vi "Read Waveform.vi"(0 "CS++Scope":refnum<class "CS++Scope.lvclass">, 1 "channel name (\"CHANNEL1\")":string="CHANNEL1", 2 "maximum time (5000ms)":i32=5000, 3 "waveform size (0)":i32=1000 caption="waveform size (1000)", 5 "error in (no error)":errorcluster) -> (14 "CS++Scope out":refnum<class "CS++Scope.lvclass">, 15 "waveform array":dbl[unit][](array[numeric]) format="%.3f", 16 "actual points":i32, 17 "initial x":dbl[unit] caption="initial x (seconds)" format="%^.2e", 18 "x increment":dbl[unit] caption="x increment (seconds)" format="%^.2e", 19 "error out":errorcluster)   [LabVIEW 2016, in "CS++Scope.lvlib" / "CS++Scope.lvclass"]
doc: "This VI initiates an acquisition on all channels that you enable with the IviScope Configure Channel VI. If the channel you specify in the Channel Name parameter is not enabled for the acquisition, this VI returns the IVISCOPE_ERROR_CHANNEL_NOT_ENABLED (0xBFFA2001) error. It then waits for the acquisition to complete and returns the waveform for the channel you specify. If the oscilloscope did not complete the acquisition within the time period you specify with the Maximum Time parameter, the VI returns the IVISCOPE_ERROR_MAX_TIME_EXCEEDED (0xBFFA2003) error.\n\nYou call the IviScope Fetch Waveform VI to obtain the waveforms for each of the remaining enabled channels without initiating another acquisition.\n\nNotes:\n \n(1) Use this VI to read waveforms when you set the acquisition mode to IVISCOPE_VAL_NORMAL, IVISCOPE_VAL_HI_RES, or IVISCOPE_VAL_AVERAGE. If the acquisition type is not one of the listed types, the VI returns the IVISCOPE_ERROR_INVALID_ACQ_TYPE (0xBFFA2004) error.\n\n(2) After this VI executes, each element in the Waveform Array parameter is either a voltage or a value indicating that the oscilloscope could not sample a voltage.\n\n(3) You configure the interpolation method the oscilloscope uses with the IviScope Is Invalid Waveform Element VI. If you disable interpolation, the oscilloscope does not interpolate points in the waveform. If the oscilloscope cannot sample a value for a point in the waveform, the driver sets the corresponding element in the Waveform Array to an IEEE defined NaN (Not a Number) value and the VI returns IVISCOPE_WARN_INVALID_WFM_ELEMENT (0x3FFA2001).\n\n(4) You can test a waveform value for an invalid value condition by calling the IviScope Is Invalid Waveform Element VI.\n\n(5) This VI performs interchangeability checking when the IviScope>>Inherent IVI Settings>>User Options>>Interchange Check property is set to TRUE. If the IviScope>>Inherent IVI Settings>>User Options>>Spy property is set to TRUE, you use the NI I/O Trace utility to view interchangeability warnings. You use the IviScope Get Next Interchange Warning VI to retrieve interchangeability warnings when the IviScope>>Inherent IVI Settings>>User Options>>Spy property is set to FALSE. For more information about interchangeability checking, refer to the help text for the IviScope>>Inherent IVI Settings>>User Options>>Interchange Check property.\n\n(6) The class driver returns a simulated waveform when this VI is called and the IviScope>>Inherent IVI Settings>>User Options>>Simulate property is set to TRUE and the IviScope>>Inherent IVI Settings>>User Options>>Use Specific Simulation property is set to FALSE. For information on how to configure a simulated waveform, refer to the online help manual."
uses:
  CS++Scope.lvclass
  CSPP_Core/Classes/CS++ProcessVariables/ProcessVariable/PV.lvclass
  PV-Enum-n.ctl
  PV-Enum.ctl
  CSPP_Core/Classes/CS++ProcessVariables/ProcessVariable/PV.lvclass/PV.ctl
  CS++Scope.lvclass/CS++Scope.ctl
  CSPP_Core/Classes/CS++ProcessVariables/ProcessVariable/Write Data.vi
  CSPP_Core/Classes/CS++ProcessVariables/ProcessVariable/Write Timestamp.vi
  CSPP_Core/Classes/CS++ProcessVariables/ProcessVariable/Write Quality.vi
  CSPP_Core/Classes/CS++ProcessVariables/ProcessVariable/Write status.vi
  CSPP_Core/Classes/CS++ProcessVariables/PVConnection/PVConnection.lvclass
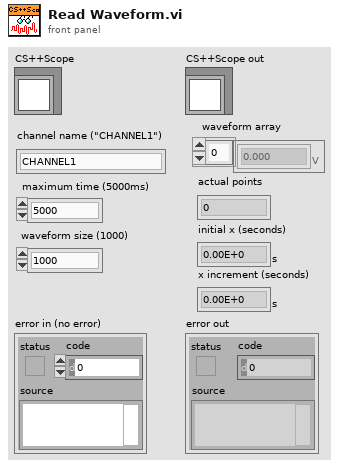
[diagram p1: front panel]
types:
  T1 = typedef "CS++Scope.lvlib/CS++Scope.lvclass/PV-Enum.ctl" = enum16{"ActualSampleRate", "TimePerRecord", "AcquisitionStartTime", "TriggerLevel", "GlitchWidth", "LowReference", "MidReference", "HighReference", "RuntLowThreshold", "RuntHighThreshold", "TriggerHoldoff", "WidthLowThreshold", "WidthHighThreshold", "AcquisitionStatus", "ActualRecordLength", "ActualSampleMode", "ACLineTriggerSlope", "MinRecordLength", "AcquisitionType", "TriggerSlope", "GlitchCondition", "GlitchPolarity", "InterpolationMethod", "NumberOfAverages", "NumberOfEnvelopes", "TriggerType", "TriggerCoupling", "TriggerModifier", "TVLineNumber", "TVEvent", "TVTriggerPolarity", "TVSignalFormat", "WidthCondition", "WidthPolarity", "MeasurementDone", "ContinousAcquisition", "TriggerSource", "Waveform", "ActualTimeIncrement"}
  T2 = typedef "CS++Scope.lvlib/CS++Scope.lvclass/PV-Enum-n.ctl" = enum16{"InputImpedance", "MaxInputFrequency", "VerticalRange", "ProbeAttenuation", "VerticalOffset", "VerticalCoupling", "ChannelEnabled"}
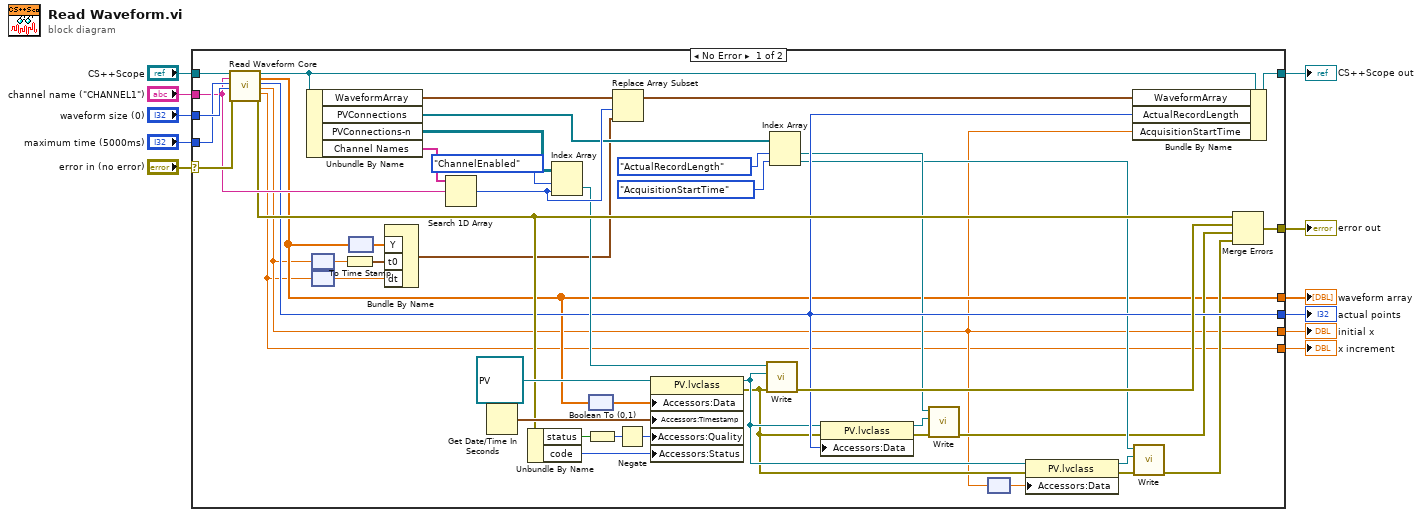
[diagram p0: block diagram]
diagram:
  n1 = case shown="No Error" "error in (no error)" {
    selector: "error in (no error)" -> [w57 w60]
    tunnel: [w40 w60] -> w10
    tunnel: [w38 w59] -> w6
    tunnel: "CS++Scope" -> [w58 w59]
    tunnel: "channel name (\"CHANNEL1\")" -> [w52 _]
    tunnel: "waveform size (0)" -> [w56 _]
    tunnel: "maximum time (5000ms)" -> [w55 _]
    tunnel: [w19 _] -> w4
    tunnel: [w13 _] -> w3
    tunnel: [w15 _] -> w2
    tunnel: [w33 _] -> w1
    frame No Error {
      n2 = call-dynamic "Read Waveform Core.vi"("CS++Scope"=w58, "channel name (\"CHANNEL1\")"=w52, "maximum time (5000ms)"=w55, "waveform size (0)"=w56, "error in (no error)"=w57) -> ("CS++Scope out"=w54:refnum<class "CS++Scope.lvclass">, "waveform array"=w19:dbl[unit][], "actual points"=w33:i32, "initial x"=w15:dbl[unit], "x increment"=w13:dbl[unit], "error out"=w43:errorcluster)  [unwired: 9 in]
      n3 = Unbundle By Name(w54) -> ("WaveformArray"=w50:waveform(dbl)[], "PVConnections"=w32:refnum<class "PVConnection.lvclass">[], "PVConnections-n"=w36:refnum<class "PVConnection.lvclass">[][], "Channel Names"=w53:string[])
      n4 = node(w15) -> (w14:dbl)
      n5 = node(w13) -> (w12:dbl)
      n6 = To Time Stamp(1:w14) -> (0:w16:timestamp)
      n7 = node(w19) -> (w17:dbl[])
      n8 = Bundle By Name("Y"=w17, "t0"=w16, "dt"=w12) -> (w18:waveform(dbl))  [unwired: 1 in]
      n9 = Search 1D Array(1D array=w53, element=w52) -> (index of element=w51:i32)  [unwired: 1 in]
      n10 = Get Date/Time In Seconds() -> (seconds since 1Jan1904=w44:timestamp)
      n11 = Unbundle By Name(w43) -> ("status"=w47:bool, "code"=w48:i32)
      n12 = Index Array(array=w36, index (row)=PV-Enum-n."ChannelEnabled" ("PV-Enum-n"), index (col)=w51) -> (element=w41:refnum<class "PVConnection.lvclass">)
      n13 = Boolean To (0,1)(Boolean=w47) -> (0, 1=w46:i16)
      n14 = node(w19) -> (w21:dbl[])
      n15 = Replace Array Subset(array=w50, new element=w18, index=w51) -> (w37:waveform(dbl)[])
      n16 = Negate(x=w46) -> (-x=w45:i16)
      n17 = property class="PV.lvclass"(reference=refnum<class "PV.lvclass"> refnum ("CS++ProcessVariables.lvlib:PV.lvclass"), "Accessors:Data"=w21, "Accessors:Timestamp"=w44, "Accessors:Quality"=w45, "Accessors:Status"=w48) -> (reference out=w26:refnum<class "PV.lvclass">, error out=w25:errorcluster)  [unwired: 1 in]
      n18 = call "Write.vi"("error in (no error)"=w25, "PV"=w26, "PVConnection in"=w41) -> ("error out"=w39:errorcluster)  [unwired: 7 in, 1 out]
      n19 = Index Array(array=w32, index #1=PV-Enum."ActualRecordLength" ("PV-Enum"), index #2=PV-Enum."AcquisitionStartTime" ("PV-Enum")) -> (element #1=w30:refnum<class "PVConnection.lvclass">, element #2=w24:refnum<class "PVConnection.lvclass">)
      n20 = property class="PV.lvclass"(reference=w26, error in=w25, "Accessors:Data"=w33) -> (reference out=w34:refnum<class "PV.lvclass">, error out=w35:errorcluster)
      n21 = call "Write.vi"("error in (no error)"=w35, "PV"=w34, "PVConnection in"=w30) -> ("error out"=w23:errorcluster)  [unwired: 7 in, 1 out]
      n22 = node(w15) -> (w20:dbl)
      n23 = property class="PV.lvclass"(reference=w26, error in=w25, "Accessors:Data"=w20) -> (reference out=w27:refnum<class "PV.lvclass">, error out=w28:errorcluster)
      n24 = Bundle By Name(cluster=w54, "WaveformArray"=w37, "ActualRecordLength"=w33, "AcquisitionStartTime"=w15) -> (w38:refnum<class "CS++Scope.lvclass">)
      n25 = call "Write.vi"("error in (no error)"=w28, "PV"=w27, "PVConnection in"=w24) -> ("error out"=w22:errorcluster)  [unwired: 7 in, 1 out]
      n26 = Merge Errors(w43, w39, w23, w22) -> (w40:errorcluster)
    }
    frame Error {
    }
  }
  "error out" <- w10
  "waveform array" <- w4
  "actual points" <- w1
  "initial x" <- w2
  "x increment" <- w3
  "CS++Scope out" <- w6
